vi "Plot Robot.vi"(6 "Length":dbl, 9 "Angle":dbl, 10 "Location":cluster{"X":dbl, "Y":dbl}, 11 "Width":dbl) -> (3 "Cluster":cluster{"X Out":dbl[], "Y Out":dbl[]})   [LabVIEW 2019, in "Pure Pursuit.lvlib"]
uses:
  Pure Pursuit.lvlib
  <vilib>/Analysis/coordinate.llb/2D Cartesian Coordinate Rotation (Array).vi
  <vilib>/Analysis/coordinate.llb/2D Cartesian Coordinate Shift (Array).vi
  <vilib>/Analysis/NI_AALPro.lvlib
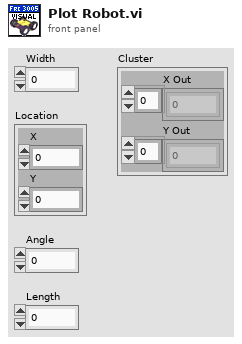
[diagram p1: front panel]
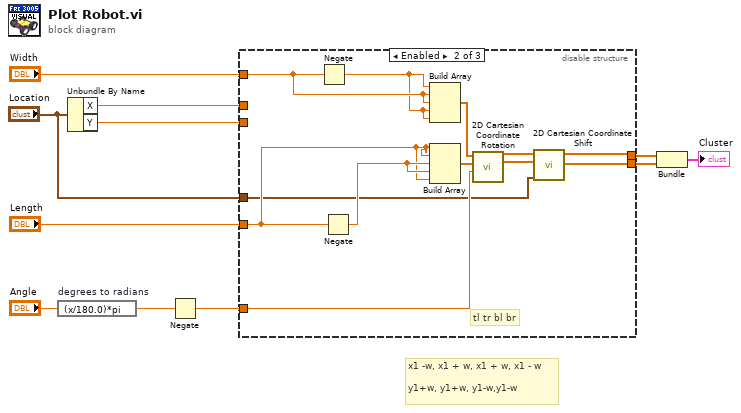
[diagram p0: block diagram]
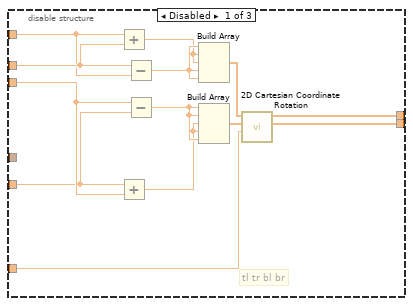
[diagram p2: hidden frame]
diagram:
  # "x1 -w, x1 + w, x1 + w, x1 - w\n\ny1+w, y1+w, y1-w,y1-w"
  n1 = expression code="(x/180.0)*pi" "degrees to radians"("Angle") -> (w10:dbl)
  n2 = Unbundle By Name("Location") -> ("X"=w3:dbl, "Y"=w5:dbl)
  n3 = Negate(x=w10) -> (-x=w11:dbl)
  n4 = disable-structure shown="Enabled" {
    disable-tunnel: w11 -> [w24 w36 _]
    disable-tunnel: [w23 w26 _] -> w8
    disable-tunnel: [w22 w25 _] -> w7
    disable-tunnel: w5 -> [w15 _ _]
    disable-tunnel: "Length" -> [w14 w32 _]
    disable-tunnel: w3 -> [w13 _ _]
    disable-tunnel: "Width" -> [w12 w35 _]
    disable-tunnel: "Location" -> [_ w27 _]
    frame Disabled {
      # "tl tr bl br"
      n5 = Add(x=w12, y=w13) -> (x+y=w16:dbl)
      n6 = Add(x=w14, y=w15) -> (x+y=w17:dbl)
      n7 = Subtract(x=w13, y=w12) -> (x-y=w19:dbl)
      n8 = Subtract(x=w15, y=w14) -> (x-y=w18:dbl)
      n9 = Build Array(w19, w16, w16, w19, w19) -> (w20:dbl[])
      n10 = Build Array(w18, w18, w17, w17, w18) -> (w21:dbl[])
      n11 = call-poly <vilib>:"2D Cartesian Coordinate Rotation.vi"("theta"=w24, "Y"=w21, "X"=w20) -> ("Y Out"=w22:dbl[], "X Out"=w23:dbl[])  [unwired: 6 in, 1 out]
    }
    frame Enabled {
      # "tl tr bl br"
      n12 = Negate(x=w35) -> (-x=w34:dbl)
      n13 = Negate(x=w32) -> (-x=w33:dbl)
      n14 = Build Array(w34, w35, w35, w34, w34) -> (w31:dbl[])
      n15 = Build Array(w32, w32, w33, w33, w32) -> (w30:dbl[])
      n16 = call-poly <vilib>:"2D Cartesian Coordinate Rotation.vi"("theta"=w36, "Y"=w30, "X"=w31) -> ("Y Out"=w28:dbl[], "X Out"=w29:dbl[])  [unwired: 6 in, 1 out]
      n17 = call-poly <vilib>:"2D Cartesian Coordinate Shift.vi"("shift"=w27, "Y"=w28, "X"=w29) -> ("Y Out"=w25:dbl[], "X Out"=w26:dbl[])  [unwired: 6 in, 1 out]
    }
    frame Disabled {
    }
  }
  n18 = Bundle("X Out"=w8, "Y Out"=w7) -> (→"Cluster":cluster{"X Out":dbl[], "Y Out":dbl[]})  [unwired: 1 in]
